vi "Opposite Direction.vi"(11 "Dir":T1) -> (3 "Opp":T1)   [LabVIEW 2020]
uses:
  Dir.ctl
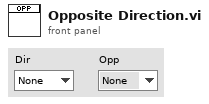
[diagram p1: front panel]
types:
  T1 = typedef "Dir.ctl" = enum16{"None", "Up", "Left", "Down", "Right"}
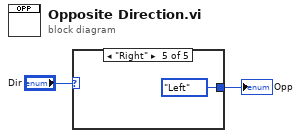
[diagram p0: block diagram]
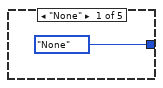
[diagram p2: hidden frame]
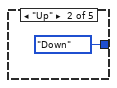
[diagram p3: hidden frame]
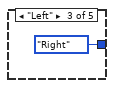
[diagram p4: hidden frame]
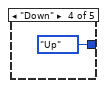
[diagram p5: hidden frame]
diagram:
  n1 = case shown="\"Right\"" "Dir" {
    tunnel: [Dir."None" ("Dir") Dir."Down" ("Dir") Dir."Right" ("Dir") Dir."Up" ("Dir") Dir."Left" ("Dir")] -> w1
    frame "None" {
    }
    frame "Up" {
    }
    frame "Left" {
    }
    frame "Down" {
    }
    frame "Right" {
    }
  }
  "Opp" <- w1
